vi "XLP80_Action_OpenCVMGUI.vi"(8 "err in":errorcluster) -> (0 "err out":errorcluster)   [LabVIEW 2021]
uses:
  XLP80_Globals/XLP80_Globals_Status.vi
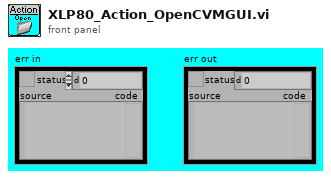
[diagram p1: front panel]
types:
  T1 = enum32{"Invalid", "Standard", "Closed", "Hidden", "Minimized", "Maximized"}
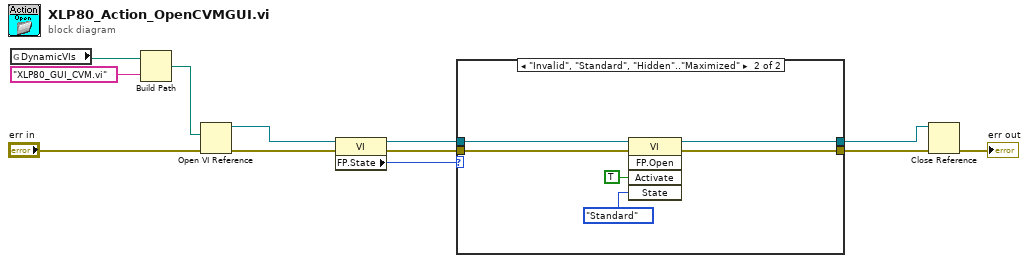
[diagram p0: block diagram]
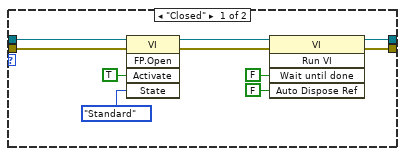
[diagram p2: hidden frame]
diagram:
  n1 = global read "XLP80_Globals_Status.vi" "DynamicVIs"() -> (w10:path)
  n2 = Build Path(base path=w10, name or relative path="XLP80_GUI_CVM.vi") -> (appended path=w8:path)
  n3 = Open VI Reference(vi path=w8, error in (no error)="err in") -> (vi reference=w1:refnum<vi>, error out=w2:errorcluster)  [unwired: 4 in]
  n4 = property class="VI"(reference=w1, error in=w2) -> (reference out=w5:refnum<vi>, error out=w4:errorcluster, "FP.State"=w3:T1)
  n5 = case shown="\"Invalid\", \"Standard\", \"Hidden\"..\"Maximized\"" w3 {
    tunnel: [w22 w23] -> w12
    tunnel: [w21 w24] -> w11
    tunnel: w5 -> [w14 w26]
    tunnel: w4 -> [w13 w25]
    frame "Closed" {
      n6 = invoke class="VI" method="FP.Open"(reference=w14, error in=w13, "Activate"=TRUE ("Activate?"), "State"=T1."Standard") -> (reference out=w18:refnum<vi>, error out=w17:errorcluster)  [unwired: 1 in, 3 out]
      n7 = invoke class="VI" method="Run VI"(reference=w18, error in=w17, "Wait until done"=FALSE ("Wait Until Done"), "Auto Dispose Ref"=FALSE ("Auto Dispose Reference")) -> (reference out=w21:refnum<vi>, error out=w22:errorcluster)  [unwired: 1 in, 3 out]
    }
    frame "Invalid", "Standard", "Hidden".."Maximized" {
      n8 = invoke class="VI" method="FP.Open"(reference=w26, error in=w25, "Activate"=TRUE ("Activate?"), "State"=T1."Standard") -> (reference out=w24:refnum<vi>, error out=w23:errorcluster)  [unwired: 1 in, 3 out]
    }
  }
  n9 = Close Reference(reference=w11, error in (no error)=w12) -> (error out=→"err out":errorcluster)
